vi "Warning.vi"() -> ()   [LabVIEW 2016]
panel:
  in  "stop":bool
  # "WARNING！SHOCK HARZARD!"
  # "Safty precautions must be taken before test!"
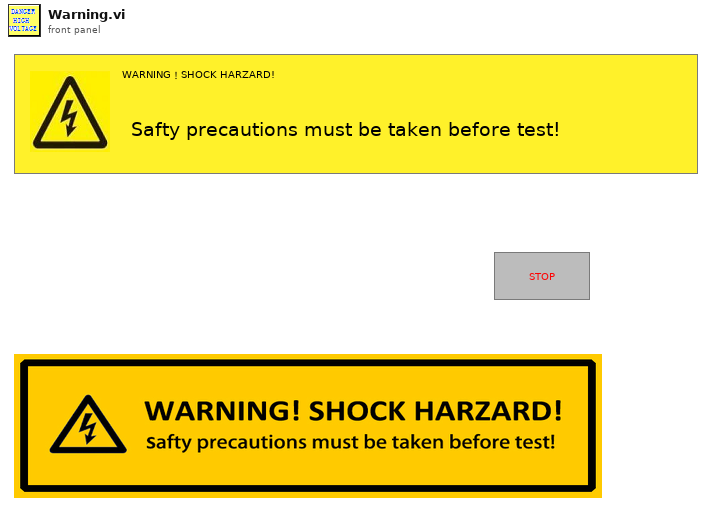
[diagram p1: front panel]
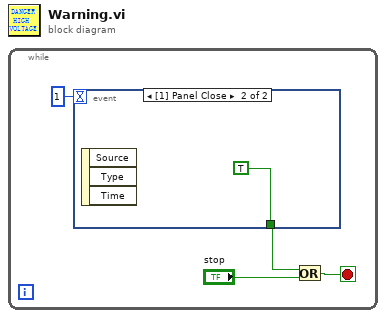
[diagram p0: block diagram]
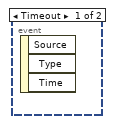
[diagram p2: hidden frame]
diagram:
  n1 = while {
    stop <- w1 stop-if-true
    n2 = event shown="[1] Panel Close" {
      selector: _ -> [_ _]
      dyn-events: _ -> [_ _]
      timeout: 1 -> [_ _]
      tunnel: [_ TRUE] -> w3
      event Timeout {
        n3 = event-data() -> ()  [unwired: 1 in, 3 out]
      }
      event Panel Close {
        n4 = event-data() -> ()  [unwired: 1 in, 3 out]
      }
    }
    n5 = Or(x=w3, y="stop") -> (x .or. y?=w1:bool)
  }
